vi "Wait Hot CMD.vi"(10 "Delay ms":u32=500) -> ()   [LabVIEW 2014]
uses:
  TORC Code/GlobalVariable.vi
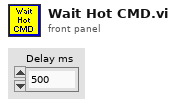
[diagram p1: front panel]
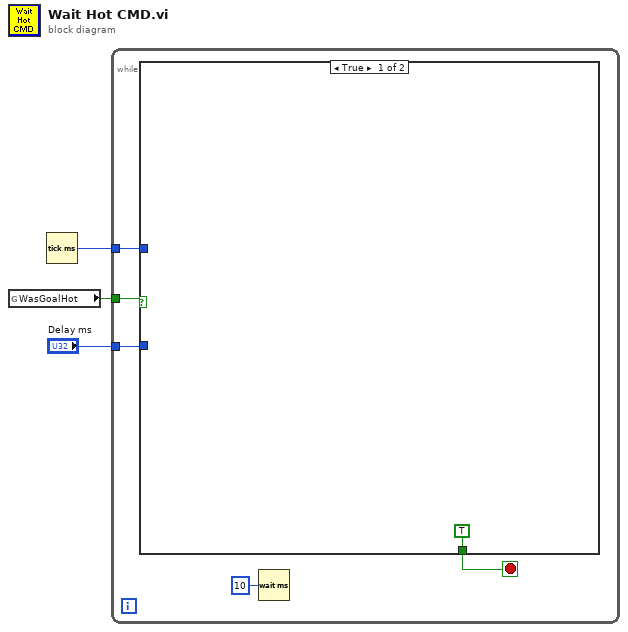
[diagram p0: block diagram]
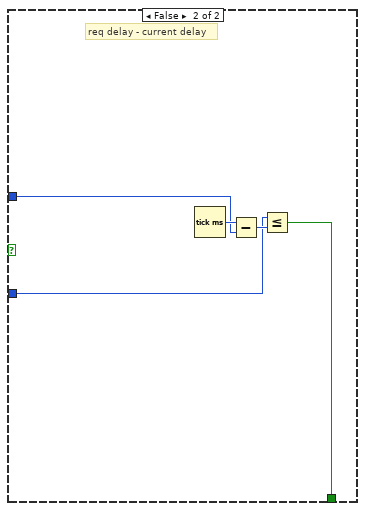
[diagram p2: hidden frame]
diagram:
  n1 = global read "GlobalVariable.vi" "WasGoalHot"() -> (w3:bool)
  n2 = Tick Count (ms)() -> (millisecond timer value=w1:u32)
  n3 = while {
    tunnel: w3 -> [w8]
    tunnel: "Delay ms" -> [w7]
    tunnel: w1 -> [w5]
    stop <- w6 stop-if-true
    n4 = case shown="True" w8 {
      tunnel: w7 -> [_ w12]
      tunnel: [TRUE w10] -> w6
      tunnel: w5 -> [_ w11]
      frame True {
      }
      frame False {
        # "req delay - current delay"
        n5 = Tick Count (ms)() -> (millisecond timer value=w13:u32)
        n6 = Subtract(x=w13, y=w11) -> (x-y=w14:u32)
        n7 = Less Or Equal?(x=w12, y=w14) -> (x <= y?=w10:bool)
      }
    }
    n8 = Wait (ms)(milliseconds to wait=u32 10 ("millisecond multiple")) -> ()  [unwired: 1 out]
  }
